vi "2D Cartesian Coordinate Shift (Array).vi"(8 "shift":cluster{"dx":dbl, "dy":dbl}, 10 "Y":dbl[](array[numeric]), 11 "X":dbl[](array[numeric])) -> (0 "error":i32, 2 "Y Out":dbl[](array[numeric]), 3 "X Out":dbl[](array[numeric]))   [LabVIEW 2020, in "NI_AALPro.lvlib"]
doc: "Shifts two-dimensional Cartesian coordinates along the x- and y-axes. Wire data to the <B>X</B> input to determine the polymorphic instance to use or manually select the instance."
uses:
  <vilib>/Analysis/NI_AALPro.lvlib
  <resource>/lvanlys.dll
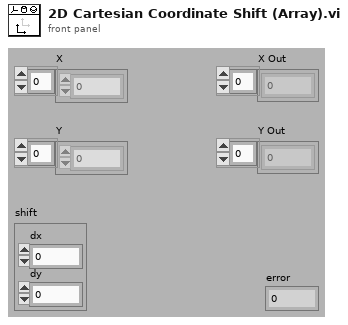
[diagram p1: front panel]
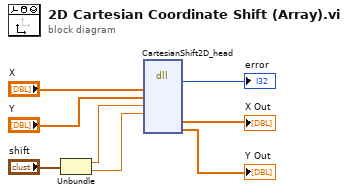
[diagram p0: block diagram]
diagram:
  n1 = Unbundle("shift") -> ("dx"=w5:dbl, "dy"=w4:dbl)
  n2 = dll-call lib="e:/builds/penguin/labview/branches/2020/dev/dist/resource/lvanlys.*" fn="CartesianShift2D_head"("X"="X", "Y"="Y", "dx"=w5, "dy"=w4) -> (→"error":i32, "Xout"=→"X Out":dbl[], "Yout"=→"Y Out":dbl[])  [unwired: 9 in, 2 out]
